vi "Config Path--constant.vi"(8 "error in (no error)":errorcluster) -> (0 "error out":errorcluster, 3 "App Config":path)   [LabVIEW 2020, in "MacroAssert.lvlib"]
doc: "Outputs the path to the config file of the tool."
uses:
  MacroAssert.lvlib
  <vilib>/Utility/sysdir.llb/System Directory Type.ctl
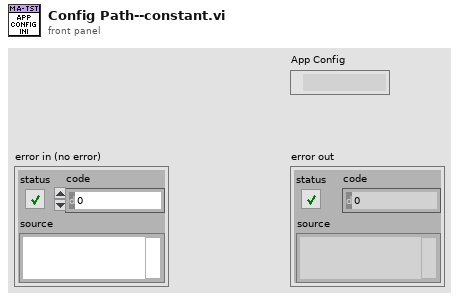
[diagram p1: front panel]
types:
  T1 = typedef "System Directory Type.ctl" = i32
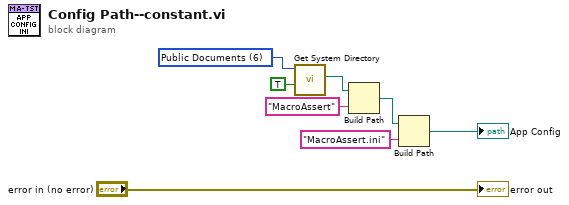
[diagram p0: block diagram]
diagram:
  w3 = T1 6 items=["User Home"=0, "User Desktop"=1, "User Documents"=2, "User Application Data"=3, "User Preferences"=4, "User Temporary"=5, "Public Documents"=6, "Public Application Data"=7, "Public Preferences"=8, "Public Cache"=13, "System Core Libraries"=9, "System Installed Libraries"=10, "Application Files"=11, "Boot Volume Root"=12] ("system directory type")
  n1 = call <vilib>:"Get System Directory.vi"("create directory if not found? (F)"=TRUE, "system directory type"=w3) -> ("system directory"=w5:path)  [unwired: 9 in]
  n2 = Build Path(base path=w5, name or relative path="MacroAssert") -> (appended path=w2:path)
  n3 = Build Path(base path=w2, name or relative path="MacroAssert.ini") -> (appended path=→"App Config":path)
  "error out" <- "error in (no error)"
